vi "Search for Main vi ref.vi"(10 "map":map{string, refnum<vi>}(c390), 11 "Child Paths Set":set{string}(c389)) -> (3 "Main vi Ref":refnum<vi>)   [LabVIEW 2020, in "Panther Dashboard.lvlib"]
uses:
  Panther Dashboard.lvlib
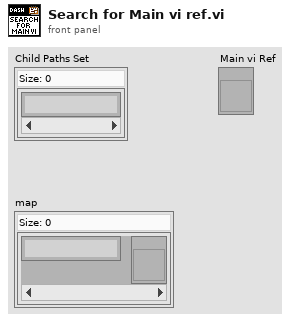
[diagram p1: front panel]
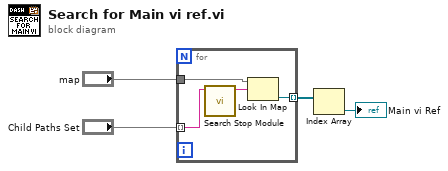
[diagram p0: block diagram]
diagram:
  n1 = for {
    tunnel: "map" -> [w8]
    tunnel: "Child Paths Set" -> [w6] mode=indexing
    tunnel: [w7] -> w3 mode=indexing
    n2 = call "Search Stop Module.vi"("Child Tree"=w6) -> ("Stop Module path"=w5:string)  [unwired: 10 in]
    n3 = Look In Map(map=w8, key=w5) -> (value=w7:refnum<vi>)  [unwired: 1 in, 1 out]
  }
  n4 = Index Array(array=w3) -> (element=→"Main vi Ref":refnum<vi>)  [unwired: 1 in]
